vi "신호시뮬레이션(열거형).vi"() -> ()   [LabVIEW 2014]
uses:
  <vilib>/Analysis/NI_AALBase.lvlib
panel:
  out "웨이브폼 그래프":dbl[](graph)
  in  "정지 버튼":bool
  in  "열거형":T1(ring)
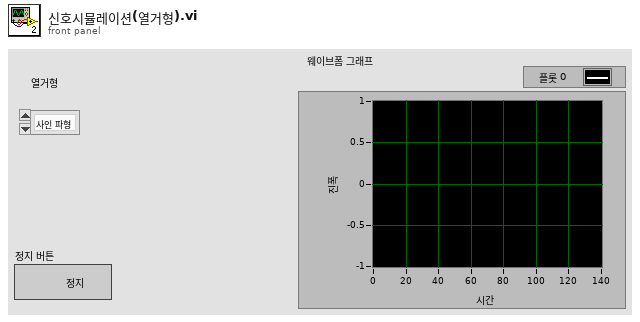
[diagram p1: front panel]
types:
  T1 = enum16{"사인 파형", "삼각 파형", "사각 파형", "톱니 파형", "노이즈"}
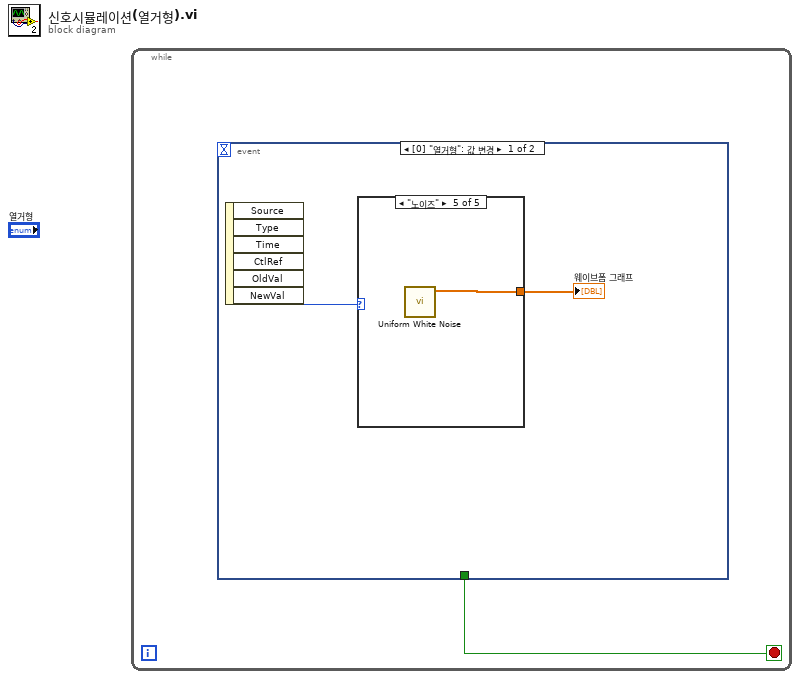
[diagram p0: block diagram]
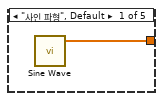
[diagram p2: hidden frame]
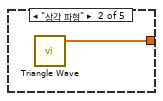
[diagram p3: hidden frame]
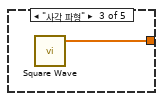
[diagram p4: hidden frame]
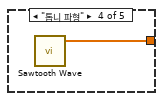
[diagram p5: hidden frame]
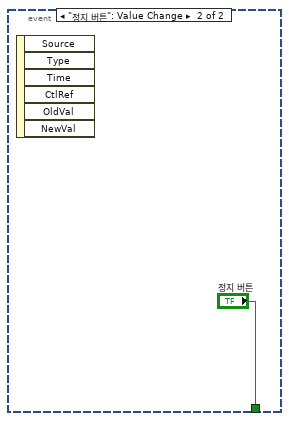
[diagram p6: hidden frame]
diagram:
  n1 = while {
    stop <- w1 stop-if-true
    n2 = event shown="[0] \"열거형\": 값 변경" {
      selector: _ -> [_ _]
      dyn-events: _ -> [_ _]
      timeout: _ -> [_ _]
      tunnel: [_ "정지 버튼"] -> w1
      event "열거형": Value Change {
        n3 = event-data() -> ("NewVal"=w3:T1)  [unwired: 1 in, 5 out]
        n4 = case shown="\"노이즈\"" w3 {
          tunnel: [w4 w5 w6 w7 w8] -> w2
          frame "사인 파형", Default {
            n5 = call <vilib>:"Sine Wave.vi"() -> ("sine wave"=w4:dbl[])  [unwired: 5 in, 2 out]
          }
          frame "삼각 파형" {
            n6 = call <vilib>:"Triangle Wave.vi"() -> ("triangle wave"=w5:dbl[])  [unwired: 5 in, 2 out]
          }
          frame "사각 파형" {
            n7 = call <vilib>:"Square Wave.vi"() -> ("square wave"=w6:dbl[])  [unwired: 6 in, 2 out]
          }
          frame "톱니 파형" {
            n8 = call <vilib>:"Sawtooth Wave.vi"() -> ("sawtooth wave"=w7:dbl[])  [unwired: 5 in, 2 out]
          }
          frame "노이즈" {
            n9 = call <vilib>:"Uniform White Noise.vi"() -> ("uniform white noise"=w8:dbl[])  [unwired: 10 in, 1 out]
          }
        }
        "웨이브폼 그래프" <- w2
      }
      event "정지 버튼": Value Change {
        n10 = event-data() -> ()  [unwired: 1 in, 6 out]
      }
    }
  }
